vi "config_text.vi"   [LabVIEW 2011]
uses:
  Main/GlobalVariables.vi
  <vilib>/regexp/Match Regular Expression.xnode
types:
  T1 = typedef "MeasureConfigType.ctl" = cluster{"Bead locations":cluster{"X":i32, "Y":i32}[], "ROI":i32, "Experiment base path":path, "Image output subdir":string, "Output mode":T2, "Traces output subdir":string, "QTrk Settings":T3, "Tracking Config":T4, "Experiment Name":string, "Program":T7, "ZLUT":sgl[][][], "Camera settings":T14, "Experiment Script":string, "Max frames in memory":i32, "Save traces as binary":bool, "Pixel Calibration Gain Image":string, "Pixel Calibration Offset Image":string, "Use pixel calibration images":bool, "Internal camera settings":string, "Trace write interval":i32}
  T2 = typedef "MeasureConfigOutputMode.ctl" = enum16{"None", "Track", "SaveImages"}
  T3 = typedef "QTrkSettings.ctl" = cluster{"Image width":i32, "Image height":i32, "Number of threads (CPU based)":i32, "CUDA Device":i32, "COM Background correction factor":sgl, "ZLUT MinRadius":sgl, "ZLUT Radial sample density":sgl, "ZLUT Angular sample density":sgl, "ZLUT ROI Coverage":sgl, "QI Iterations":i32, "QI MinRadius":sgl, "QI Radial sample density":sgl, "QI Angular sample density":sgl, "QI ROI Coverage":sgl, "QI Angular Step \nIteration Factor":sgl, "XCOR Profile Length":i32, "XCOR Profile Width":i32, "XCOR Iterations":i32, "Gaussian 2D Fit Iterations":i32, "Gaussian 2D Sigma (pixels)":sgl, "Downsample":i32}
  T4 = typedef "TrackingConfigType.ctl" = cluster{"Number of steps":i32, "ZLUT stepsize (um)":sgl, "Z correction factor":sgl, "Start piezo Z (um)":sgl, "Pixel size (nm)":sgl, "2D Localization Type":T5, "Z Command (None)":T6, "Z Piezo scale":bool, "ZLUT Building\nimages per frame":i32, "ZLUT Bias correction planes":i32}
  T5 = typedef "QTrkLocalizationType.ctl" = enum16{"Center-of-Mass", "1D Cross-Correlation", "Quadrant Interpolation", "Gaussian 2D MLE", "QI + ZLUTAlign", "ZLUTAlign", "QI + FourierLUT"}
  T6 = typedef "QTrkZCommandType.ctl" = enum16{"Nothing", "ComputeZ", "BuildRadialZLUT", "BuildImageZLUT", "RadialZLUT+ImageZLUT"}
  T7 = typedef "ExperimentProgramType.ctl" = cluster{"Commands":T8[], "Motor Axis accuracy conditions":T11, "Axis flags":T13}
  T8 = typedef "ExProgCommandType.ctl" = cluster{"cmd":T9, "axis":T10, "value/pos":dbl, "speed":dbl, "name":string}
  T9 = typedef "ExProgCommandEnumType.ctl" = enum16{"wait", "move", "event", "idle", "when", "section", "stop"}
  T10 = typedef "MotorAxisEnum.ctl" = enum16{"no axis", "magrot", "magpos", "px", "py", "pz", "camx", "camy"}
  T11 = typedef "MotorPosType.ctl" = cluster{"Magnet Z":dbl, "Magnet rotation":dbl, "Camera":T12, "Piezo XY":T12, "Piezo Z":dbl}
  T12 = typedef "XYf.ctl" = cluster{"X":sgl, "Y":sgl}
  T13 = typedef "MotorPosFlagsType.ctl" = cluster{"Magnet Z":bool, "Magnet rotation":bool, "Camera":cluster{"X":bool, "Y":bool}, "Piezo XY":cluster{"X":bool, "Y":bool}, "Piezo Z":bool}
  T14 = typedef "GenericCameraConfigType.ctl" = cluster{"Framerate (Hz)":i32, "Exposure time (us)":i32, "Image size":cluster{"Width":i32, "Height":i32}, "Number of buffers":i32}
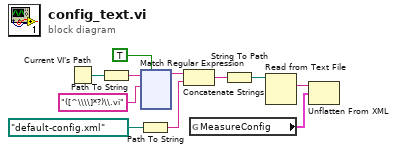
[diagram p0: block diagram]
diagram:
  n1 = Current VI's Path() -> (path=w11:path)
  n2 = Path To String(path=w11) -> (string=w10:string)
  n3 = Path To String(path=path "default-config.xml" ("file (use dialog)")) -> (string=w3:string)
  n4 = xnode "Match Regular Expression"("input string"=w10, "regular expression"="([^\\\\]*?)\\.vi", "ignore case? (F)"=TRUE) -> ("before match"=w4:string)  [unwired: 3 in, 4 out]
  n5 = Concatenate Strings(w4, w3) -> (w2:string)
  n6 = global read "GlobalVariables.vi" "MeasureConfig"() -> (w6:T1)
  n7 = String To Path(string=w2) -> (path=w1:path)
  n8 = Read from Text File(file (use dialog)=w1) -> (text=w7:string)  [unwired: 3 in, 3 out]
  n9 = Unflatten From XML(xml string=w7, type=w6) -> ()  [unwired: 1 in, 2 out]
